vi "Main.vi"() -> ()   [LabVIEW 2020, in "Application.lvlib"]
doc: "This VI is the main application VI in the DQMH project template. This application VI is implemented as a simple state machine, which communicates with two different DQMH modules.\n_____\nBased on DQMH Dev Tools: Project Template 7.1.2.1547."
uses:
  Application.lvlib
  Application Data--cluster.ctl
  DAQ AI/DAQ AI.lvlib
  UI/UI.lvlib
  State--enum.ctl
  <vilib>/Utility/error.llb/DialogType.ctl
panel:
  in  "About DQMH":bool
  out "version":string
  in  "Hide UI Module":bool
  in  "Show UI Module":bool
  in  "Hide DAQ AI Module":bool
  in  "Show DAQ AI Module":bool
  in  "Stop DAQ AI Module":bool
  in  "Stop UI Module":bool
  in  "Start UI Module":bool
  out "Active DAQ AI Modules":string[](array[string])
  in  "Start New Instance DAQ AI Module":bool
  in  "Select DAQ AI Module Instance":i32(ring)=-1 items=["All"=-1]
  out "UI Running?":bool
  out "Status":string
  # "This top-level application allows you to launch and control a singleton module, and multiple instances of a cloneable module."
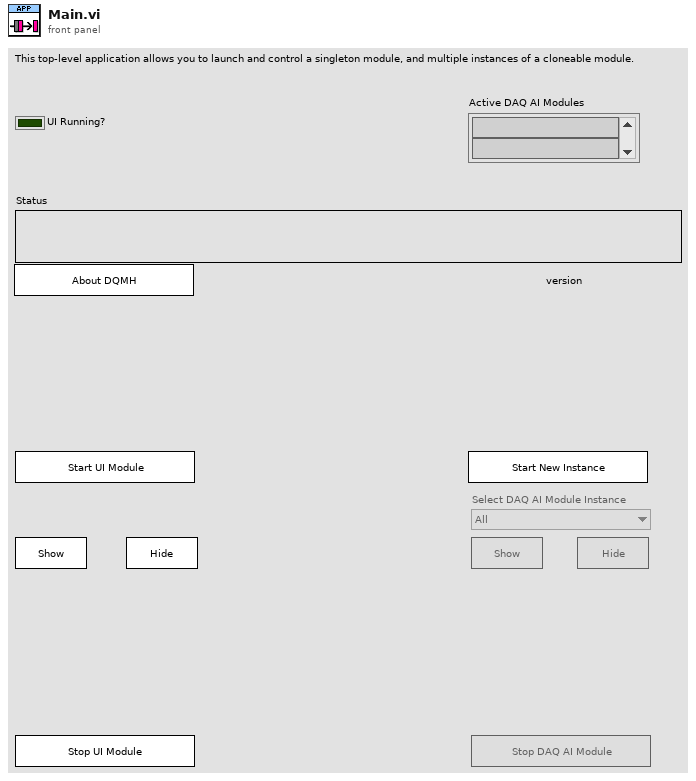
[diagram p1: front panel]
types:
  T1 = typedef "Application.lvlib/State--enum.ctl" = enum16{"Initialize", "Initialize Panel", "UI Interlocks", "Launch UI Module", "Update Status", "Wait for Event", "Start Acquisition", "Stop Acquisition", "Error", "Exit"}
  T2 = typedef "Application.lvlib/Application Data--cluster.ctl" = cluster{"Status":string, "Singleton Controls":refnum<vi>[], "Cloneable Controls":refnum<vi>[], "Module Ring Value":i32, "Acquiring":bool, "DAQmx Analog Channels":tag[], "Close Flag":bool}
  T3 = typedef "DAQ AI.lvlib/Broadcast Events--cluster.ctl" = cluster{"Module Did Init":refnum<user-event>, "Status Updated":refnum<user-event>, "Error Reported":refnum<user-event>, "Module Did Stop":refnum<user-event>, "Update Module Execution Status":refnum<user-event>, "Send Acquired Data":refnum<user-event>, "Clear DAQ Task":refnum<user-event>}
  T4 = typedef "UI.lvlib/Broadcast Events--cluster.ctl" = cluster{"Module Did Init":refnum<user-event>, "Status Updated":refnum<user-event>, "Error Reported":refnum<user-event>, "Module Did Stop":refnum<user-event>, "Update Module Execution Status":refnum<user-event>, "Start Acquisition":refnum<user-event>, "Stop Acquisition":refnum<user-event>, "Close":refnum<user-event>}
  T5 = enum8{"Enabled", "Disabled", "Disabled and Grayed Out"}
  T6 = typedef "DialogType.ctl" = u16
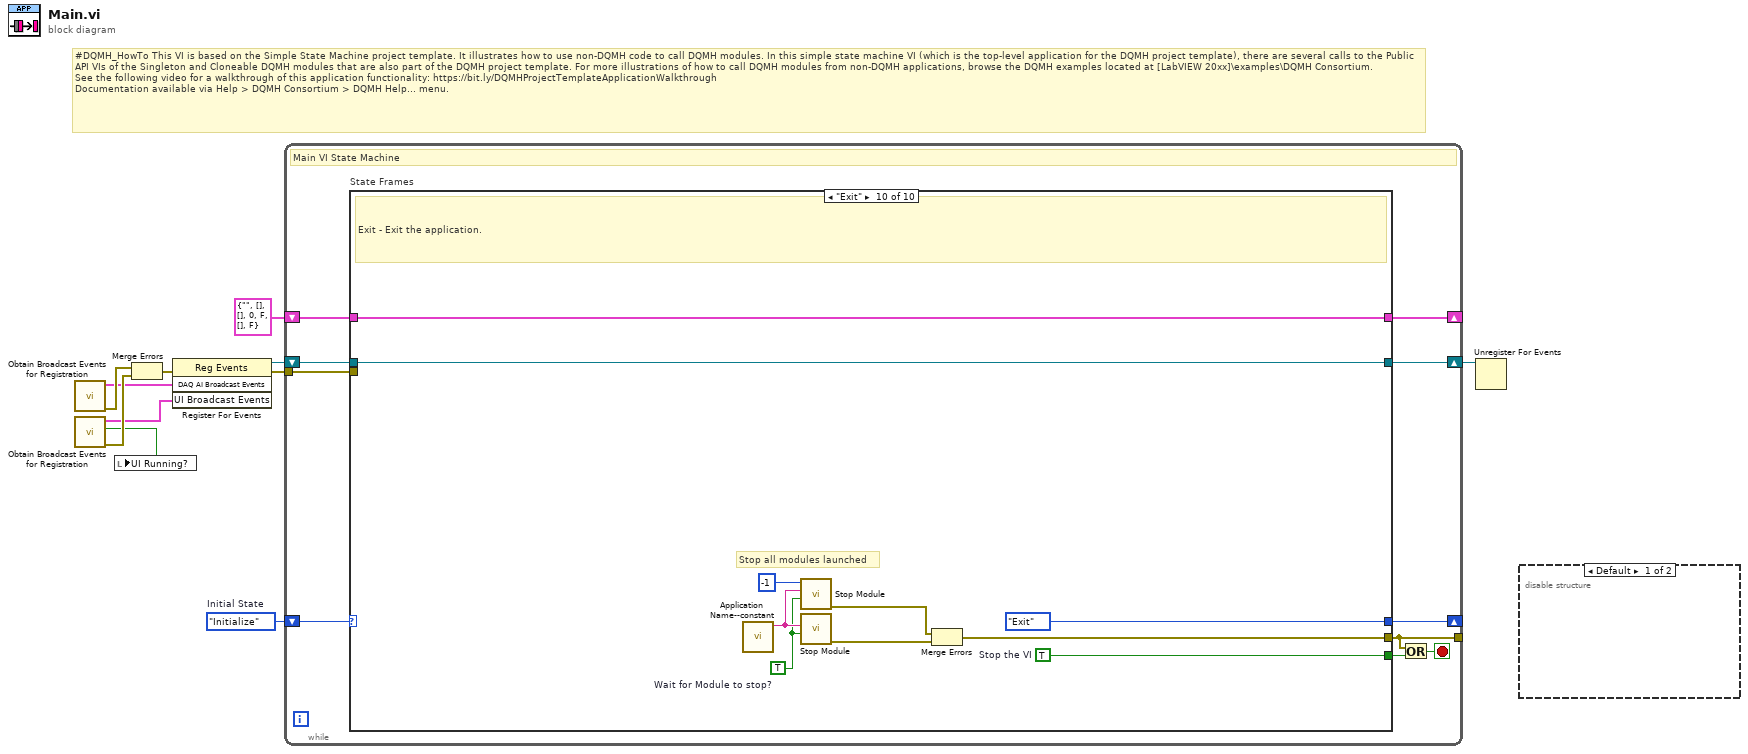
[diagram p0: block diagram]
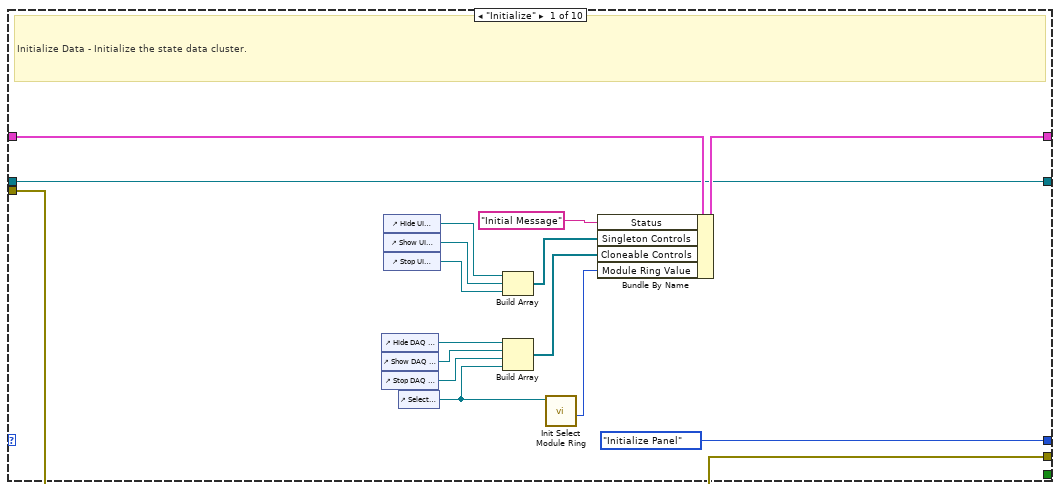
[diagram p2: hidden frame]
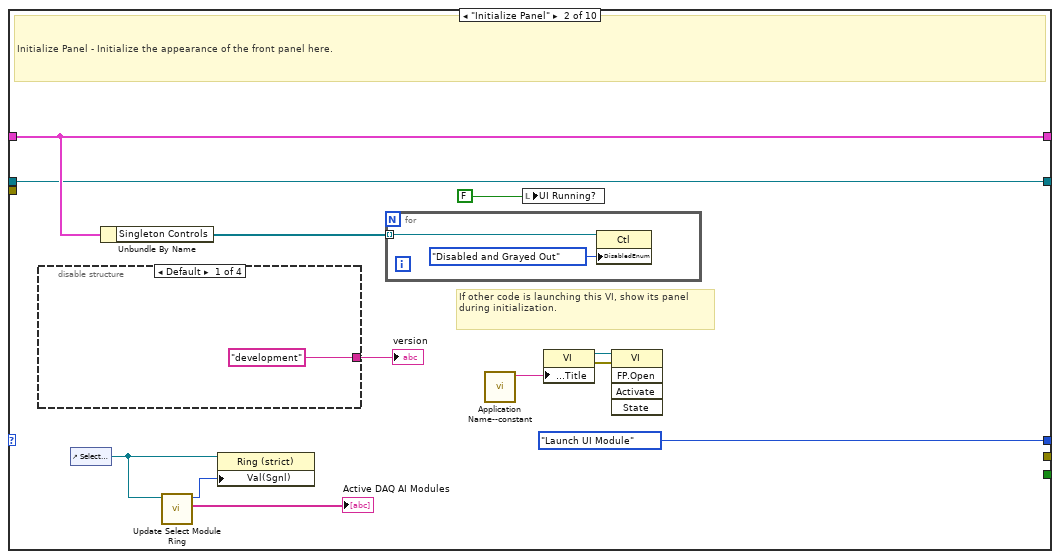
[diagram p3: hidden frame]
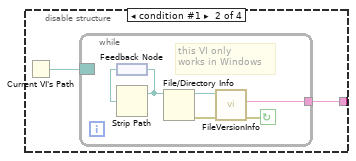
[diagram p4: hidden frame]
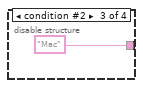
[diagram p5: hidden frame]
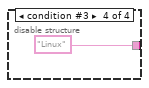
[diagram p6: hidden frame]
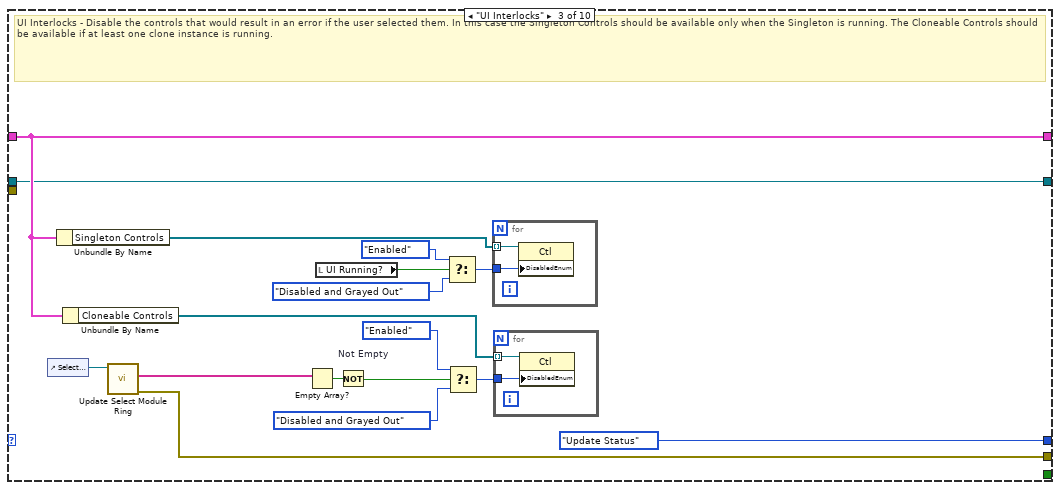
[diagram p7: hidden frame]
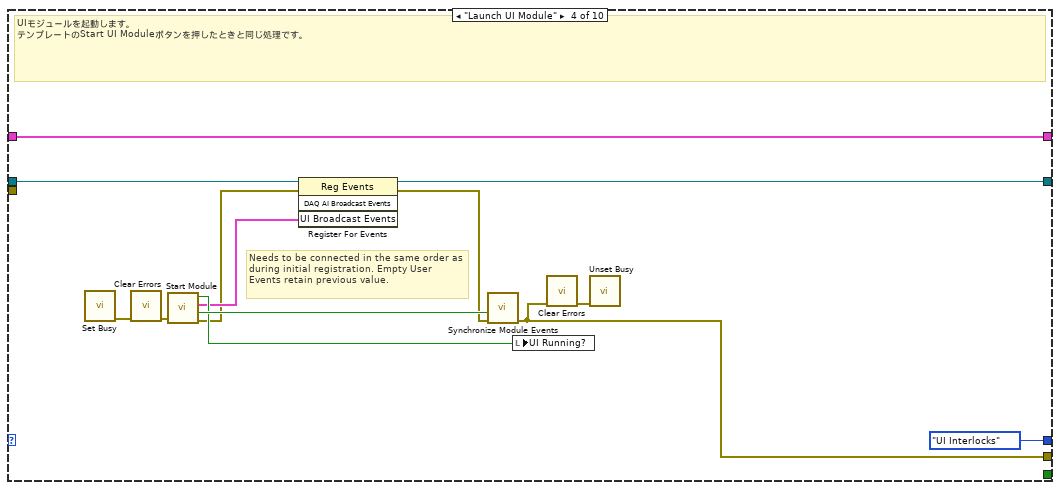
[diagram p8: hidden frame]
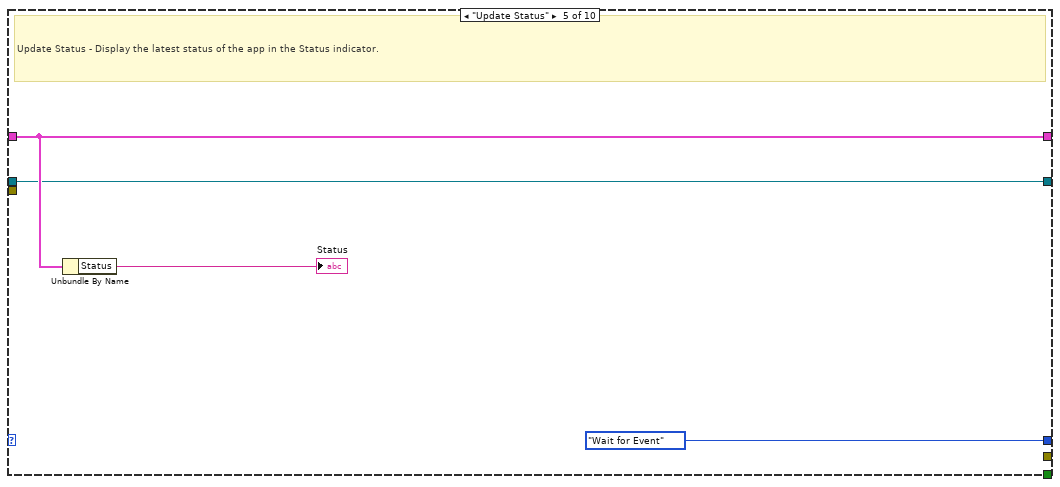
[diagram p9: hidden frame]
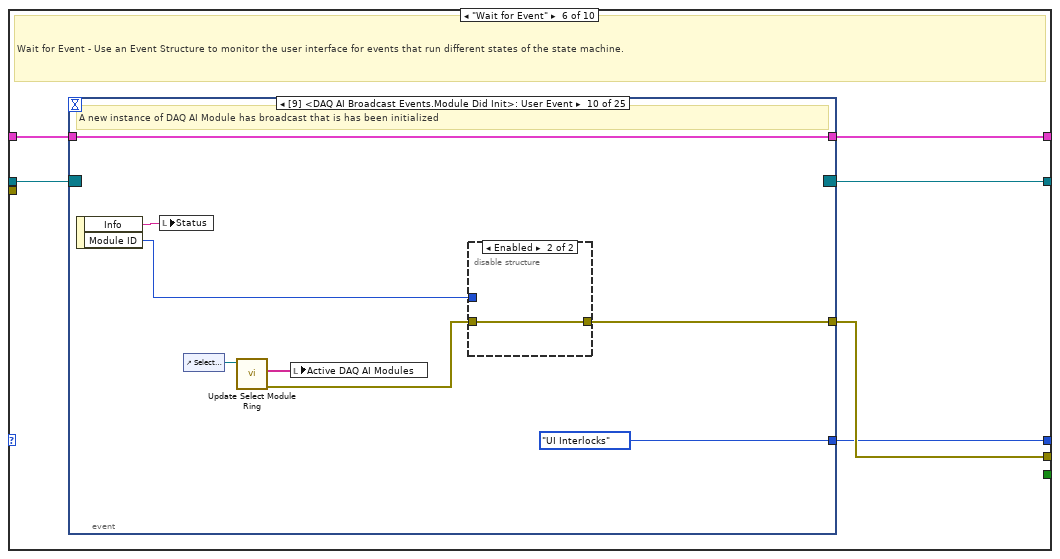
[diagram p10: hidden frame]
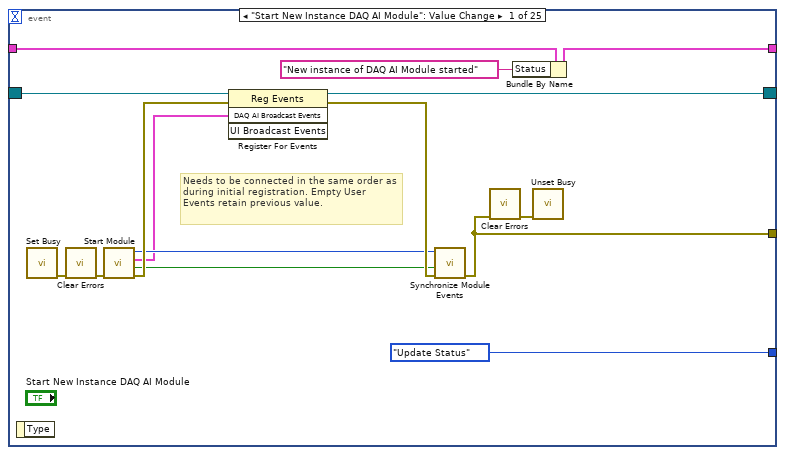
[diagram p11: hidden frame]
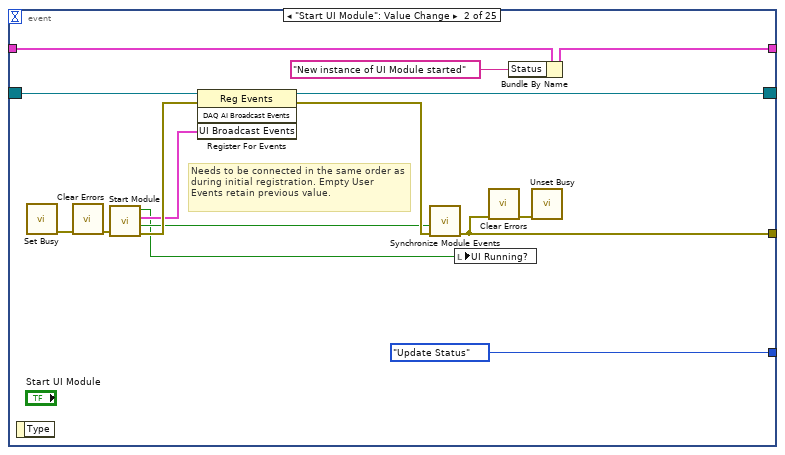
[diagram p12: hidden frame]
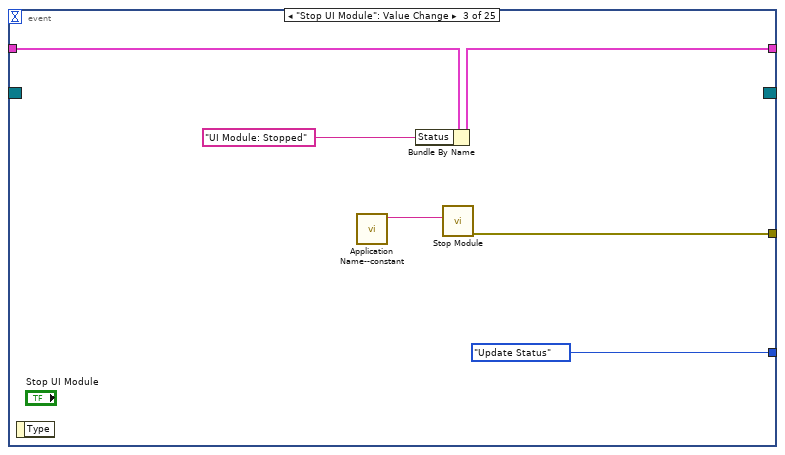
[diagram p13: hidden frame]
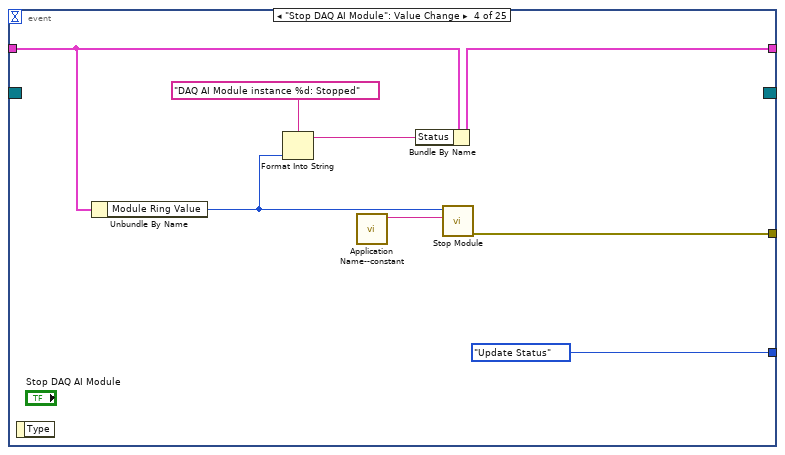
[diagram p14: hidden frame]
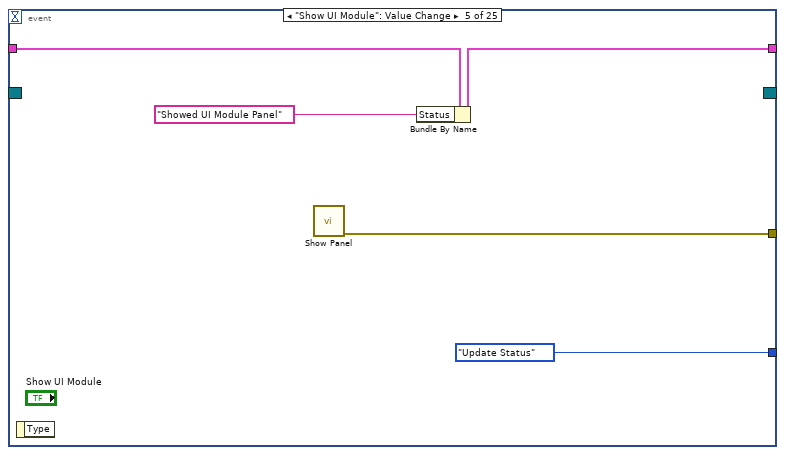
[diagram p15: hidden frame]
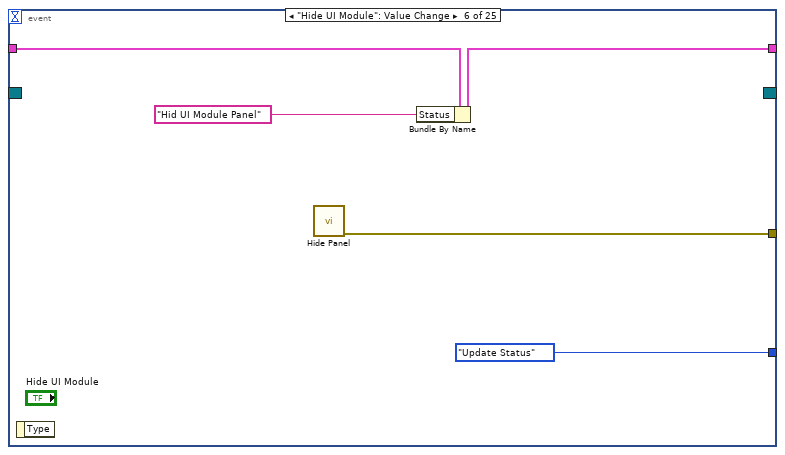
[diagram p16: hidden frame]
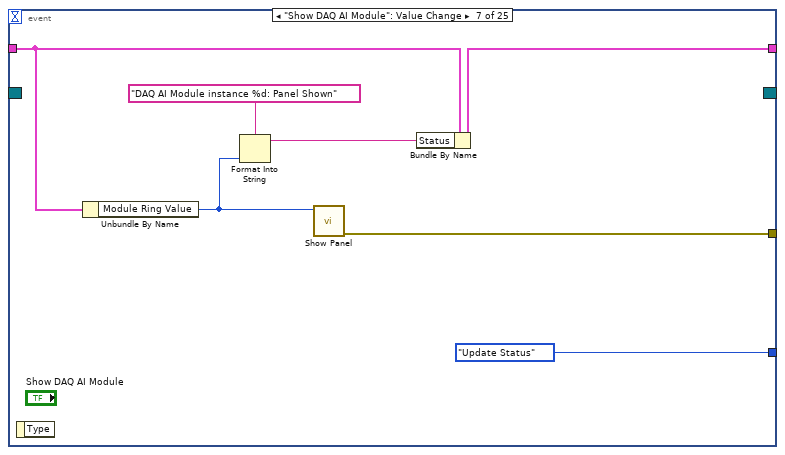
[diagram p17: hidden frame]
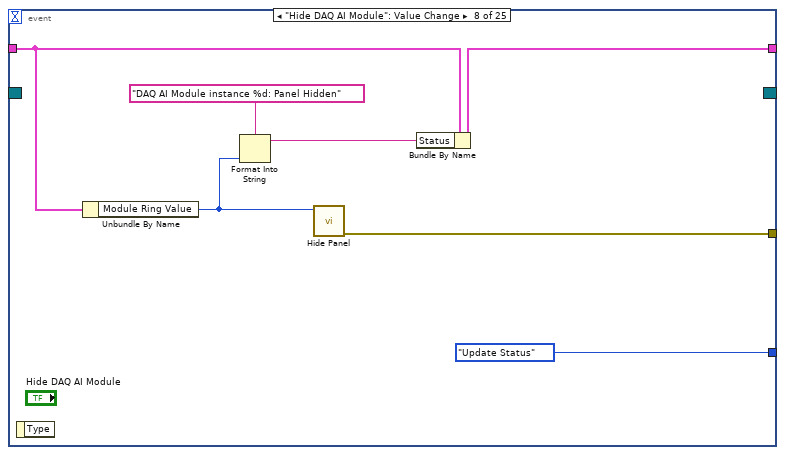
[diagram p18: hidden frame]
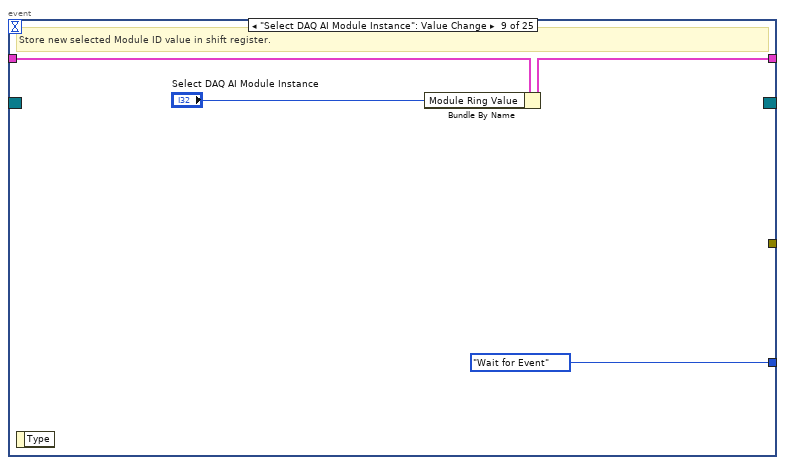
[diagram p19: hidden frame]
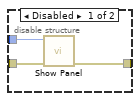
[diagram p20: hidden frame]
diagram:
  w4 = State--enum."Initialize"  # Initial State
  # "#DQMH_HowTo This VI is based on the Simple State Machine project template. It illustrates how to use non-DQMH code to call DQMH modules. In this simple state machine VI (which is the top-level application for the DQMH project template), there are several calls to the Public API VIs of the Singleton and Cloneable DQMH modules that are also part of the DQMH project template. For more illustrations of how to call DQMH modules from non-DQMH applications, browse the DQMH examples located at [LabVIEW 20xx]\\examples\\DQMH Consortium.\nSee the following video for a walkthrough of this application functionality: https://bit.ly/DQMHProjectTemplateApplicationWalkthrough\nDocumentation available via Help > DQMH Consortium > DQMH Help... menu."
  n1 = call "Obtain Broadcast Events for Registration.vi"() -> ("error out"=w9:errorcluster, "DAQ AI Broadcast Events"=w6:T3)  [unwired: 9 in, 1 out]
  n2 = call "Obtain Broadcast Events for Registration.vi"() -> ("error out"=w8:errorcluster, "Already running?"=w1:bool, "UI Broadcast Events"=w5:T4)  [unwired: 9 in]
  n3 = local write "UI Running?"(w1) -> ()
  n4 = Merge Errors(w9, w8) -> (w10:errorcluster)
  n5 = register-events(error in=w10, w6, w5) -> (reference out=w3:refnum<event-registration>, error out=w11:errorcluster)  [unwired: 1 in]
  n6 = while {
    shift-right: [w18] -> _
    shift-left: T2 {"Status"="", "Singleton Controls"=[], "Cloneable Controls"=[], "Module Ring Value"=0, "Acquiring"=FALSE, "DAQmx Analog Channels"=[], "Close Flag"=FALSE} ("Data Cluster") -> [w19]
    tunnel: [w21] -> _
    shift-right: [w14] -> _
    shift-left: w4 -> [w16]
    shift-right: [w12] -> w2
    shift-left: w3 -> [w13]
    tunnel: w11 -> [w20]
    stop <- w15 stop-if-true
    # "Main VI State Machine"
    n7 = case "State Frames" shown="\"Exit\"" w16 {
      tunnel: [w37 _ w79 w84 _ w106 w291 w321 _ w345] -> w21
      tunnel: w19 -> [w36 w46 w67 w96 w100 w103 w293 w325 w331 w342]
      tunnel: [w35 w46 w67 w96 w100 w102 w292 w324 w330 w342] -> w18
      tunnel: [_ _ _ _ _ _ _ _ _ w341] -> w17
      tunnel: [State--enum."Initialize Panel" ("State") State--enum."Launch UI Module" ("State") State--enum."Update Status" ("State") State--enum."UI Interlocks" ("State") State--enum."Wait for Event" ("State") w101 State--enum."Wait for Event" ("State") State--enum."Wait for Event" ("State") State--enum."Exit" ("State") State--enum."Exit" ("State")] -> w14
      tunnel: w13 -> [w22 w43 w63 w94 w97 w105 w301 w322 w335 w339]
      tunnel: [w22 w43 w63 w93 w97 w104 w294 w322 w335 w339] -> w12
      tunnel: w20 -> [w37 _ _ _ _ _ _ _ _ _]
      frame "Initialize" {
        # "Initialize Data - Initialize the state data cluster."
        n8 = control-ref of="Hide DAQ AI Module"() -> (w29:refnum<vi>)
        n9 = control-ref of="Show DAQ AI Module"() -> (w28:refnum<vi>)
        n10 = control-ref of="Stop DAQ AI Module"() -> (w27:refnum<vi>)
        n11 = control-ref of="Hide UI Module"() -> (w33:refnum<vi>)
        n12 = control-ref of="Show UI Module"() -> (w32:refnum<vi>)
        n13 = control-ref of="Stop UI Module"() -> (w31:refnum<vi>)
        n14 = control-ref of="Select DAQ AI Module Instance"() -> (w24:refnum<vi>)
        n15 = Build Array(w33, w32, w31) -> (w30:refnum<vi>[])
        n16 = Build Array(w29, w28, w27, w24) -> (w26:refnum<vi>[])
        n17 = call "Init Select Module Ring.vi"("Select Module Ring Ref"=w24) -> ("Module Ring Value"=w23:i32)  [unwired: 8 in, 2 out]
        n18 = Bundle By Name(cluster=w36, "Status"="Initial Message" ("Initial Message"), "Singleton Controls"=w30, "Cloneable Controls"=w26, "Module Ring Value"=w23) -> (w35:T2)
      }
      frame "Initialize Panel" {
        # "If other code is launching this VI, show its panel during initialization."
        # "Initialize Panel - Initialize the appearance of the front panel here."
        n19 = disable-structure "Conditional Disable Structure" shown="Default" {
          disable-tunnel: ["development" w51 "Mac" "Linux"] -> w40
          frame condition #0 (active) {
          }
          frame condition #1 {
            n20 = Current VI's Path() -> (path=w52:path)
            n21 = while {
              border: w52 -> [_]
              tunnel: [w53] -> w51
              stop <- w57 continue-if-true
              # "this VI only \nworks in Windows"
              n22 = feedback #1() -> (w56:path)
              n23 = Strip Path(path=w56) -> (stripped path=w55:path)  [unwired: 1 out]
              n24 = feedback-in #1(w55) -> ()
              n25 = File/Directory Info(path=w55) -> (path out=w54:path, error out=w58:errorcluster)  [unwired: 1 in, 5 out]
              n26 = call <vilib>:"FileVersionInfo.vi"("error in (no error)"=w58, "Application Path in"=w54) -> ("error out"=w57:errorcluster, "File Version Info"=w53:string)  [unwired: 6 in, 2 out]
            }
          }
          frame condition #2 {
          }
          frame condition #3 {
          }
        }
        "version" <- w40
        n27 = control-ref of="Select DAQ AI Module Instance"() -> (w42:refnum<vi>)
        n28 = Unbundle By Name(w46) -> ("Singleton Controls"=w45:refnum<vi>[])
        n29 = call "Update Select Module Ring.vi"("Select Module Ring Ref"=w42) -> ("Active Modules (Array)"=→"Active DAQ AI Modules":string[], "New Module Ring Value"=w41:i32)  [unwired: 8 in, 1 out]
        n30 = property on="Property Node" class="Ring (strict)"(reference=w42, "Val(Sgnl)"=w41) -> ()  [unwired: 1 in, 2 out]
        n31 = for {
          tunnel: w45 -> [w62] mode=indexing
          n32 = property on="Property Node" class="Ctl"(reference=w62, "DisabledEnum"=T5."Disabled and Grayed Out" ("Disabled")) -> ()  [unwired: 1 in, 2 out]
        }
        n33 = call "Application Name--constant.vi"() -> ("Application Name"=w39:string)  [unwired: 11 in]
        n34 = local write "UI Running?"(FALSE ("My Singleton Module Init?")) -> ()
        n35 = property on="Property Node" class="VI"("Front Panel.Title"=w39) -> (reference out=w38:refnum<vi>, error out=w49:errorcluster)  [unwired: 2 in]
        n36 = invoke class="VI" method="FP.Open"(reference=w38, error in=w49) -> ()  [unwired: 3 in, 5 out]
      }
      frame "UI Interlocks" {
        # "UI Interlocks - Disable the controls that would result in an error if the user selected them. In this case the Singleton Controls should be available only when the Singleton is running. The Cloneable Controls should be available if at least one clone instance is running."
        n37 = control-ref of="Select DAQ AI Module Instance"() -> (w78:refnum<vi>)
        n38 = Unbundle By Name(w67) -> ("Singleton Controls"=w72:refnum<vi>[])
        n39 = Unbundle By Name(w67) -> ("Cloneable Controls"=w66:refnum<vi>[])
        n40 = call "Update Select Module Ring.vi"("Select Module Ring Ref"=w78) -> ("error out"=w79:errorcluster, "Active Modules (Array)"=w77:string[])  [unwired: 8 in, 1 out]
        n41 = Empty Array?(array=w77) -> (empty?=w76:bool)
        n42 = local read "UI Running?"() -> (w71:bool)
        n43 = Not "Not Empty"(x=w76) -> (.not. x?=w65:bool)
        n44 = Select(t=T5."Enabled" ("Disabled"), s=w71, f=T5."Disabled and Grayed Out" ("Disabled")) -> (s? t:f=w73:T5)
        n45 = Select(t=T5."Enabled" ("Disabled"), s=w65, f=T5."Disabled and Grayed Out" ("Disabled")) -> (s? t:f=w70:T5)
        n46 = for {
          tunnel: w72 -> [w83] mode=indexing
          tunnel: w73 -> [w82]
          n47 = property on="Property Node" class="Ctl"(reference=w83, "DisabledEnum"=w82) -> ()  [unwired: 1 in, 2 out]
        }
        n48 = for {
          tunnel: w66 -> [w81] mode=indexing
          tunnel: w70 -> [w80]
          n49 = property on="Property Node" class="Ctl"(reference=w81, "DisabledEnum"=w80) -> ()  [unwired: 1 in, 2 out]
        }
      }
      frame "Launch UI Module" {
        # "Needs to be connected in the same order as during initial registration. Empty User Events retain previous value."
        # "UIモジュールを起動します。\nテンプレートのStart UI Moduleボタンを押したときと同じ処理です。"
        n50 = call <vilib>:"Set Busy.vi"() -> ("error out"=w91:errorcluster)  [unwired: 10 in, 1 out]
        n51 = call <vilib>:"Clear Errors.vi"("error in (no error)"=w91) -> ("error out"=w92:errorcluster)  [unwired: 5 in, 1 out]
        n52 = call "Start Module.vi"("error in"=w92) -> ("error out"=w86:errorcluster, "Wait for Event Sync?"=w89:bool, "UI Broadcast Events"=w87:T4, "Module Was Already Running?"=w88:bool)  [unwired: 6 in, 1 out]
        n53 = register-events(reference=w94, error in=w86, w87) -> (reference out=w93:refnum<event-registration>, error out=w85:errorcluster)  [unwired: 1 in]
        n54 = call "Synchronize Module Events.vi"("error in"=w85, "Wait for Event Sync?"=w89) -> ("error out"=w84:errorcluster)  [unwired: 9 in]
        n55 = local write "UI Running?"(w88) -> ()
        n56 = call <vilib>:"Clear Errors.vi"("error in (no error)"=w84) -> ("error out"=w90:errorcluster)  [unwired: 5 in, 1 out]
        n57 = call <vilib>:"Unset Busy.vi"("error in (no error)"=w90) -> ()  [unwired: 10 in, 1 out]
      }
      frame "Update Status" {
        # "Update Status - Display the latest status of the app in the Status indicator."
        n58 = Unbundle By Name(w100) -> ("Status"=→"Status":string)
      }
      frame "Wait for Event" {
        # "Wait for Event - Use an Event Structure to monitor the user interface for events that run different states of the state machine."
        n59 = event shown="[9] <DAQ AI Broadcast Events.Module Did Init>: User Event" {
          selector: w105 -> [w113 w129 _ _ _ _ _ _ _ _ _ _ _ _ _ _ _ _ _ _ _ _ _ _ _]
          dyn-events: [w112 w128 _ _ _ _ _ _ _ _ _ _ _ _ _ _ _ _ _ _ _ _ _ _ _] -> w104
          timeout: _ -> [_ _ _ _ _ _ _ _ _ _ _ _ _ _ _ _ _ _ _ _ _ _ _ _ _]
          tunnel: [w121 w136 w142 w150 w155 w160 w167 w174 _ w186 w195 w199 _ _ _ _ w241 _ _ w255 _ _ _ w278 w288] -> w106
          tunnel: [w108 w125 w138 w147 w153 w158 w166 w173 w176 w180 w192 w198 w201 w206 w221 w230 w234 w245 w250 w257 w258 w263 w269 w279 w289] -> w102
          tunnel: w103 -> [w109 w126 w139 w146 w154 w159 w164 w171 w177 w180 w192 w198 w202 w207 w222 w231 w237 w246 w250 w257 w260 w263 w268 w279 w284]
          tunnel: [State--enum."Update Status" ("State") State--enum."Update Status" ("State") State--enum."Update Status" ("State") State--enum."Update Status" ("State") State--enum."Update Status" ("State") State--enum."Update Status" ("State") State--enum."Update Status" ("State") State--enum."Update Status" ("State") State--enum."Wait for Event" ("State") State--enum."UI Interlocks" ("State") State--enum."UI Interlocks" ("State") State--enum."UI Interlocks" ("State") State--enum."Update Status" ("State") State--enum."Update Status" ("State") State--enum."Error" ("State") State--enum."Error" ("State") State--enum."UI Interlocks" ("State") State--enum."UI Interlocks" ("State") w251 State--enum."Wait for Event" ("State") State--enum."Start Acquisition" ("State") State--enum."Stop Acquisition" ("State") w264 State--enum."Wait for Event" ("State") w280] -> w101
          event "Start New Instance DAQ AI Module": Value Change {
            # "Needs to be connected in the same order as during initial registration. Empty User Events retain previous value."
            n60 = event-data() -> ()  [unwired: 1 in, 1 out]
            n61 = call <vilib>:"Set Busy.vi"() -> ("error out"=w117:errorcluster)  [unwired: 10 in, 1 out]
            n62 = call <vilib>:"Clear Errors.vi"("error in (no error)"=w117) -> ("error out"=w118:errorcluster)  [unwired: 5 in, 1 out]
            n63 = call "Start Module.vi"("error in"=w118) -> ("error out"=w120:errorcluster, "Wait for Event Sync?"=w115:bool, "DAQ AI Broadcast Events"=w111:T3, "Module ID"=w114:i32)  [unwired: 6 in, 1 out]
            n64 = register-events(reference=w113, error in=w120, w111) -> (reference out=w112:refnum<event-registration>, error out=w119:errorcluster)  [unwired: 1 in]
            n65 = call "Synchronize Module Events.vi"("error in"=w119, "Wait for Event Sync?"=w115, "Module ID in"=w114) -> ("error out"=w121:errorcluster)  [unwired: 7 in, 1 out]
            n66 = call <vilib>:"Clear Errors.vi"("error in (no error)"=w121) -> ("error out"=w116:errorcluster)  [unwired: 5 in, 1 out]
            n67 = Bundle By Name(cluster=w109, "Status"="New instance of DAQ AI Module started") -> (w108:T2)
            n68 = call <vilib>:"Unset Busy.vi"("error in (no error)"=w116) -> ()  [unwired: 10 in, 1 out]
          }
          event "Start UI Module": Value Change {
            # "Needs to be connected in the same order as during initial registration. Empty User Events retain previous value."
            n69 = event-data() -> ()  [unwired: 1 in, 1 out]
            n70 = call <vilib>:"Set Busy.vi"() -> ("error out"=w132:errorcluster)  [unwired: 10 in, 1 out]
            n71 = call <vilib>:"Clear Errors.vi"("error in (no error)"=w132) -> ("error out"=w133:errorcluster)  [unwired: 5 in, 1 out]
            n72 = call "Start Module.vi"("error in"=w133) -> ("error out"=w135:errorcluster, "Wait for Event Sync?"=w130:bool, "UI Broadcast Events"=w123:T4, "Module Was Already Running?"=w122:bool)  [unwired: 6 in, 1 out]
            n73 = register-events(reference=w129, error in=w135, w123) -> (reference out=w128:refnum<event-registration>, error out=w134:errorcluster)  [unwired: 1 in]
            n74 = call "Synchronize Module Events.vi"("error in"=w134, "Wait for Event Sync?"=w130) -> ("error out"=w136:errorcluster)  [unwired: 9 in]
            n75 = local write "UI Running?"(w122) -> ()
            n76 = call <vilib>:"Clear Errors.vi"("error in (no error)"=w136) -> ("error out"=w131:errorcluster)  [unwired: 5 in, 1 out]
            n77 = Bundle By Name(cluster=w126, "Status"="New instance of UI Module started") -> (w125:T2)
            n78 = call <vilib>:"Unset Busy.vi"("error in (no error)"=w131) -> ()  [unwired: 10 in, 1 out]
          }
          event "Stop UI Module": Value Change {
            n79 = event-data() -> ()  [unwired: 1 in, 1 out]
            n80 = call "Application Name--constant.vi"() -> ("Application Name"=w140:string)  [unwired: 11 in]
            n81 = Bundle By Name(cluster=w139, "Status"="UI Module: Stopped" ("Message")) -> (w138:T2)
            n82 = call "Stop Module.vi"("Origin"=w140) -> ("error out"=w142:errorcluster)  [unwired: 10 in]
          }
          event "Stop DAQ AI Module": Value Change {
            n83 = event-data() -> ()  [unwired: 1 in, 1 out]
            n84 = Unbundle By Name(w146) -> ("Module Ring Value"=w143:i32)
            n85 = Format Into String(format string="DAQ AI Module instance %d: Stopped" ("Message"), w143) -> (resulting string=w144:string)  [unwired: 2 in, 1 out]
            n86 = call "Application Name--constant.vi"() -> ("Application Name"=w148:string)  [unwired: 11 in]
            n87 = Bundle By Name(cluster=w146, "Status"=w144) -> (w147:T2)
            n88 = call "Stop Module.vi"("Origin"=w148, "Module ID"=w143) -> ("error out"=w150:errorcluster)  [unwired: 9 in]
          }
          event "Show UI Module": Value Change {
            n89 = event-data() -> ()  [unwired: 1 in, 1 out]
            n90 = call "Show Panel.vi"() -> ("error out"=w155:errorcluster)  [unwired: 11 in]
            n91 = Bundle By Name(cluster=w154, "Status"="Showed UI Module Panel" ("Message")) -> (w153:T2)
          }
          event "Hide UI Module": Value Change {
            n92 = event-data() -> ()  [unwired: 1 in, 1 out]
            n93 = call "Hide Panel.vi"() -> ("error out"=w160:errorcluster)  [unwired: 11 in]
            n94 = Bundle By Name(cluster=w159, "Status"="Hid UI Module Panel" ("Message")) -> (w158:T2)
          }
          event "Show DAQ AI Module": Value Change {
            n95 = event-data() -> ()  [unwired: 1 in, 1 out]
            n96 = Unbundle By Name(w164) -> ("Module Ring Value"=w162:i32)
            n97 = Format Into String(format string="DAQ AI Module instance %d: Panel Shown" ("Message"), w162) -> (resulting string=w161:string)  [unwired: 2 in, 1 out]
            n98 = call "Show Panel.vi"("Module ID"=w162) -> ("error out"=w167:errorcluster)  [unwired: 10 in]
            n99 = Bundle By Name(cluster=w164, "Status"=w161) -> (w166:T2)
          }
          event "Hide DAQ AI Module": Value Change {
            n100 = event-data() -> ()  [unwired: 1 in, 1 out]
            n101 = Unbundle By Name(w171) -> ("Module Ring Value"=w169:i32)
            n102 = Format Into String(format string="DAQ AI Module instance %d: Panel Hidden" ("Message"), w169) -> (resulting string=w168:string)  [unwired: 2 in, 1 out]
            n103 = call "Hide Panel.vi"("Module ID"=w169) -> ("error out"=w174:errorcluster)  [unwired: 10 in]
            n104 = Bundle By Name(cluster=w171, "Status"=w168) -> (w173:T2)
          }
          event "Select DAQ AI Module Instance": Value Change {
            # "Store new selected Module ID value in shift register."
            n105 = event-data() -> ()  [unwired: 1 in, 1 out]
            n106 = Bundle By Name(cluster=w177, "Module Ring Value"="Select DAQ AI Module Instance") -> (w176:T2)
          }
          event User Event {
            # "A new instance of DAQ AI Module has broadcast that is has been initialized"
            n107 = event-data() -> ("Info"=w184:string, "Module ID"=w179:i32)  [unwired: 1 in]
            n108 = local write "Status"(w184) -> ()
            n109 = control-ref of="Select DAQ AI Module Instance"() -> (w183:refnum<vi>)
            n110 = call "Update Select Module Ring.vi"("Select Module Ring Ref"=w183) -> ("error out"=w185:errorcluster, "Active Modules (Array)"=w182:string[])  [unwired: 8 in, 1 out]
            n111 = local write "Active DAQ AI Modules"(w182) -> ()
            n112 = disable-structure shown="Enabled" {
              disable-tunnel: [w189 w190] -> w186
              disable-tunnel: w185 -> [w188 w190]
              disable-tunnel: w179 -> [w187 _]
              frame Disabled {
                n113 = call "Show Panel.vi"("error in"=w188, "Module ID"=w187) -> ("error out"=w189:errorcluster)  [unwired: 9 in]
              }
              frame Enabled {
              }
            }
          }
          event User Event {
            # "UI Module has broadcast that it has been initialized"
            n114 = event-data() -> ("Init?"=→"UI Running?":bool, "Info"=w194:string)  [unwired: 1 in]
            n115 = local write "Status"(w194) -> ()
            n116 = call "Show Panel.vi"() -> ("error out"=w195:errorcluster)  [unwired: 11 in]
          }
          event User Event {
            # "UI Module has broadcast its execution status"
            n117 = event-data() -> ("Running?"=w196:bool)  [unwired: 1 in]
            n118 = local write "UI Running?"(w196) -> ()
            n119 = case shown="True" w196 {
              tunnel: [_ w200] -> w199
              frame False {
              }
              frame True {
                n120 = call "Show Panel.vi"() -> ("error out"=w200:errorcluster)  [unwired: 11 in]
              }
            }
          }
          event User Event {
            # "An instance of DAQ AI Module has broadcast its status"
            n121 = event-data() -> ("Status"=w204:string)  [unwired: 1 in]
            n122 = Bundle By Name(cluster=w202, "Status"=w204) -> (w201:T2)
          }
          event User Event {
            # "UI Module has broadcast its status"
            n123 = event-data() -> ("Status"=w208:string)  [unwired: 1 in]
            n124 = Bundle By Name(cluster=w207, "Status"=w208) -> (w206:T2)
          }
          event User Event {
            w213 = T6 0 items=["no dialog", "OK message", "continue or stop message", "OK message + warnings", "continue/stop + warnings"] ("type of dialog (OK msg:1)")
            # "DAQ AI Module had an error"
            n125 = event-data() -> ("Module Name"=w210:string, "Additional Information"=w211:string, "Error"=w212:errorcluster)  [unwired: 1 in]
            n126 = call <vilib>:"Space Constant.vi"() -> ("String"=w217:string)
            n127 = call <vilib>:"Simple Error Handler.vi"("type of dialog (OK msg:1)"=w213, "error in (no error)"=w212) -> ("message"=w214:string)  [unwired: 3 in, 4 out]
            n128 = call <vilib>:"Search and Replace Pattern.vi"("string"=w214, "regular expression (\"\")"="[\\r\\n]" ("regular expression (\"\")"), "replace string (\"\")"=w217, "replace all? (F)"=TRUE ("replace all CR/LF with spaces")) -> ("result string"=w215:string)  [unwired: 1 in, 1 out]
            n129 = Format Into String(format string="%s: %s Additional Information: %s", w210, w215, w211) -> (resulting string=w209:string)  [unwired: 2 in, 1 out]
            n130 = Bundle By Name(cluster=w222, "Status"=w209) -> (w221:T2)
          }
          event User Event {
            # "UI Module had an error"
            n131 = event-data() -> ("Module Name"=w224:string, "Additional Information"=w228:string, "Error"=w232:errorcluster)  [unwired: 1 in]
            n132 = Unbundle By Name(w232) -> ("code"=w223:i32, "source"=w227:string)
            n133 = Format Into String(format string="Error code %d Module: %s  Additional Information: %s\nSource: %s", w223, w224, w228, w227) -> (resulting string=w225:string)  [unwired: 2 in, 1 out]
            n134 = Bundle By Name(cluster=w231, "Status"=w225) -> (w230:T2)
          }
          event User Event {
            n135 = event-data() -> ("Origin"=w236:string)  [unwired: 1 in]
            n136 = Bundle By Name(cluster=w237, "Status"=w236) -> (w235:T2)
            n137 = control-ref of="Select DAQ AI Module Instance"() -> (w240:refnum<vi>)
            n138 = call "Update Select Module Ring.vi"("Select Module Ring Ref"=w240) -> ("error out"=w241:errorcluster, "Active Modules (Array)"=w239:string[], "New Module Ring Value"=w233:i32)  [unwired: 8 in]
            n139 = Bundle By Name(cluster=w235, "Module Ring Value"=w233) -> (w234:T2)
            n140 = local write "Active DAQ AI Modules"(w239) -> ()
          }
          event User Event {
            n141 = event-data() -> ("Origin"=w243:string)  [unwired: 1 in]
            n142 = local write "UI Running?"(FALSE ("My Singleton Module Init?")) -> ()
            n143 = Concatenate Strings(w243, " Did Stop.") -> (w242:string)
            n144 = Bundle By Name(cluster=w246, "Status"=w242) -> (w245:T2)
          }
          event Panel Close? {
            # "Go to the 'Exit' state if the user tries to close the panel."
            n145 = event-data() -> ()  [unwired: 1 in, 1 out]
            n146 = Unbundle By Name(w250) -> ("Acquiring"=w249:bool)
            n147 = Select(t=State--enum."Stop Acquisition" ("State"), s=w249, f=State--enum."Exit" ("State")) -> (s? t:f=w251:T1)
            n148 = event-data ("Event Filter Node")("Discard?"=TRUE) -> ()  [unwired: 1 in, 1 out]
          }
          event "About DQMH": Value Change {
            # "Display DQMH About Box"
            n149 = event-data() -> ()  [unwired: 1 in, 1 out]
            n150 = call <vilib>:"DQMH_About Box.vi"() -> ("error out"=w255:errorcluster)  [unwired: 11 in]
          }
          event User Event {
            # "UIモジュールからStart Acquisitionを受け取る"
            n151 = event-data() -> ("DAQmx Analog Channels"=w259:tag[])  [unwired: 1 in]
            n152 = Bundle By Name(cluster=w260, "DAQmx Analog Channels"=w259) -> (w258:T2)
          }
          event User Event {
            n153 = event-data() -> ()  [unwired: 1 in, 5 out]
          }
          event User Event {
            # "アプリケーション終了をUIから受け取ったときの処理"
            n154 = event-data() -> ()  [unwired: 1 in, 5 out]
            n155 = Unbundle By Name(w268) -> ("Acquiring"=w267:bool)
            n156 = Select(t=State--enum."Stop Acquisition" ("State"), s=w267, f=State--enum."Exit" ("State")) -> (s? t:f=w264:T1)
            n157 = Bundle By Name(cluster=w268, "Close Flag"=TRUE) -> (w269:T2)
          }
          event User Event {
            # "データをUIに送る"
            # "DAQ AIモジュールがデータを取得したときの処理"
            n158 = event-data() -> ("Module ID"=w272:i32, "Value"=w276:dbl)  [unwired: 1 in]
            n159 = control-ref of="Select DAQ AI Module Instance"() -> (w275:refnum<vi>)
            n160 = call "Update Select Module Ring.vi"("Select Module Ring Ref"=w275) -> ("Active Modules (Array)"=w274:string[])  [unwired: 8 in, 2 out]
            n161 = Decimal String To Number(string=w274) -> (number=w273:i32[])  [unwired: 2 in, 1 out]
            n162 = Search 1D Array(1D array=w273, element=w272) -> (index of element=w271:i32)  [unwired: 1 in]
            n163 = call "Get Analog Data.vi"("Value"=w276, "Index"=w271) -> ("error out"=w278:errorcluster)  [unwired: 9 in]
          }
          event User Event {
            # "DAQタスクをクリアした時の処理"
            n164 = event-data() -> ()  [unwired: 1 in, 1 out]
            n165 = Unbundle By Name(w284) -> ("Close Flag"=w281:bool)
            n166 = call "Application Name--constant.vi"() -> ("Application Name"=w286:string)  [unwired: 11 in]
            n167 = call "Stop Module.vi"("Origin"=w286, "Module ID"=-1) -> ("error out"=w288:errorcluster)  [unwired: 9 in]
            n168 = Select(t=State--enum."Exit" ("State"), s=w281, f=State--enum."Wait for Event" ("State")) -> (s? t:f=w280:T1)
            n169 = Bundle By Name(cluster=w284, "DAQmx Analog Channels"=tag[] []) -> (w289:T2)
          }
        }
      }
      frame "Start Acquisition" {
        # "すべてのモジュール起動後に\nDAQ物理チャンネルと\n集録周期を送る"
        # "集録開始の処理をします。\nまず、DAQ AIモジュールを起動します。\nその後、DAQ物理チャンネルと集録周期を送ります。"
        n170 = Unbundle By Name(w293) -> ("DAQmx Analog Channels"=w295:tag[])
        n171 = Array Size(array=w295) -> (size(s)=w298:i32)
        n172 = for {
          N: w298 -> [_]
          shift-right: [w312] -> w294
          shift-left: w301 -> [w313]
          shift-right: [w311] -> w297
          shift-left: errorcluster {"status"=FALSE, "code"=0, "source"=""} ("error out") -> [w310]
          tunnel: [w309] -> w296 mode=indexing
          # "モジュールを起動"
          # "Needs to be connected in the same order as during initial registration. Empty User Events retain previous value."
          n173 = call "Start Module.vi"("error in"=w310) -> ("error out"=w318:errorcluster, "Wait for Event Sync?"=w316:bool, "DAQ AI Broadcast Events"=w314:T3, "Module ID"=w315:i32)  [unwired: 6 in, 1 out]
          n174 = register-events(reference=w313, error in=w318, w314) -> (reference out=w312:refnum<event-registration>, error out=w317:errorcluster)  [unwired: 1 in]
          n175 = call "Synchronize Module Events.vi"("error in"=w317, "Wait for Event Sync?"=w316, "Module ID in"=w315) -> ("error out"=w311:errorcluster, "Module ID out"=w309:i32)  [unwired: 7 in]
        }
        n176 = for {
          shift-right: [w304] -> w291
          shift-left: w297 -> [w308]
          tunnel: w296 -> [w306] mode=indexing
          tunnel: w295 -> [w307] mode=indexing
          n177 = call "Get DAQ Analog Channel.vi"("error in"=w308, "DAQmx Physical Channel"=w307, "Module ID"=w306) -> ("error out"=w305:errorcluster)  [unwired: 8 in]
          n178 = call "Get Acquisition Period.vi"("error in"=w305, "Period [ms]"=100, "Module ID"=w306) -> ("error out"=w304:errorcluster)  [unwired: 8 in]
          n179 = Wait Until Next ms Multiple(millisecond multiple=u32 1000) -> ()  [unwired: 1 out]
        }
        n180 = Not(x=w291) -> (.not. x?=w290:bool)
        n181 = Bundle By Name(cluster=w293, "Acquiring"=w290) -> (w292:T2)
      }
      frame "Stop Acquisition" {
        # "すべてのモジュールに集録終了を送る"
        # "集録停止の処理をします。"
        n182 = Bundle By Name(cluster=w325, "Acquiring"=FALSE) -> (w324:T2)
        n183 = call "Stop Acquisition.vi"("Dummy"=TRUE, "Module ID"=-1) -> ("error out"=w321:errorcluster)  [unwired: 9 in]
      }
      frame "Error" {
        # "モジュールでエラーが発生した時の処理"
        n184 = Unbundle By Name(w331) -> ("Status"=w334:string)
        n185 = call <vilib>:"Error Cluster From Error Code.vi"("error message (\"\")"=w334, "error code (0)"=5000 ("error code (no error:0)")) -> ("error out"=w332:errorcluster)  [unwired: 7 in]
        n186 = call <vilib>:"Simple Error Handler.vi"("error in (no error)"=w332) -> ()  [unwired: 4 in, 5 out]
        n187 = Bundle By Name(cluster=w331, "Close Flag"=TRUE, "Acquiring"=FALSE) -> (w330:T2)
      }
      frame "Exit" {
        w336 = TRUE  # Wait for Module to stop?
        w341 = TRUE  # Stop the VI
        # "Stop all modules launched"
        # "Exit - Exit the application."
        n188 = call "Application Name--constant.vi"() -> ("Application Name"=w337:string)  [unwired: 11 in]
        n189 = call "Stop Module.vi"("Wait for Module to stop? (F)"=w336, "Origin"=w337, "Module ID"=-1) -> ("error out"=w343:errorcluster)  [unwired: 8 in]
        n190 = call "Stop Module.vi"("Wait for Module to Stop? (F)"=w336, "Origin"=w337) -> ("error out"=w344:errorcluster)  [unwired: 9 in]
        n191 = Merge Errors(w343, w344) -> (w345:errorcluster)
      }
    }
    n192 = Or(x=w21, y=w17) -> (x .or. y?=w15:bool)
  }
  n193 = Unregister For Events(event registration refnum=w2) -> ()  [unwired: 1 in, 1 out]
  n194 = disable-structure "Conditional Disable Structure" shown="Default" {
    frame condition #0 (active) {
    }
    frame condition #1 {
      # "Call Quit LabVIEW if running as a built application."
      n195 = Quit LabVIEW() -> ()  [unwired: 1 in]
    }
  }
